vi "CAN.vi"() -> ()   [LabVIEW 2020]
uses:
  Global_Variable/Global.vi
  Global_Variable/A180648.vi
  Libraries/ZLG_CAN/ZLG_CAN.lvlib
panel:
  out "error out":errorcluster caption="错误输出"
  in  "CAN 通道":u32(ring) items=["0", "1"]
  in  "索引":u32(ring) items=["0", "1", "2", "3", "4", "5", "6", "7", "8"]
  in  "设备类型":u32(ring)=27 items=["PCI5121"=1, "PCI9810"=2, "USBCAN1"=3, "USBCAN2"=4, "PCI9820"=5, "PCI5110"=7, "PC104CAN"=11, "CANETUDP"=12, "PCI9840B"=14, "PC104C2"=15, "PCI9820I"=16, "CANETTCP"=17, "PCIE9221"=24, "PCI5010U"=19, "USBCAN_E_U"=20, "USBCAN_2E_U"=21, "PCI5020U"=22, "PCIE9120I"=27, "PCIE9110I"=28, "PCIE9140I"=29]
  in  "Stop":bool
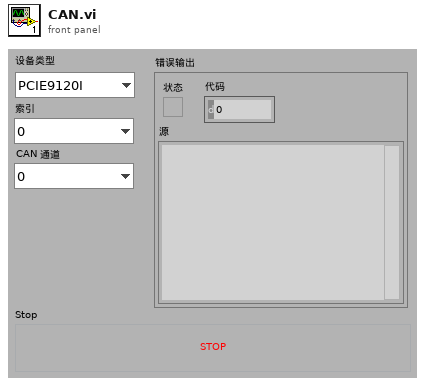
[diagram p1: front panel]
types:
  T1 = cluster{"波特率":u32, "ID":u32, "帧类型":enum8{"标准帧", "扩展帧"}, "帧格式":enum16{"数据帧", "远程帧"}, "周期(ms)":u32}
  T2 = typedef "ZLG_CAN.lvlib/Start_CAN (Reply Payload)--cluster.ctl" = cluster{"Success":bool, "Start_CAN_error":errorcluster}
  T3 = cluster{u8, u8, "y":u8, "y":u8, "y":u8, "y":u8, "y":u8, "y":u8}
  T4 = cluster{"y":u8, "y":u8, "y":u8, u8, u8, "y":u8, "y":u8, "y":u8}
  T5 = cluster{"[0]":u8, "[1]":u8, "[2]":u8, "[3]":u8, "[4]":u8, "[5]":u8, "[6]":u8, "[7]":u8}
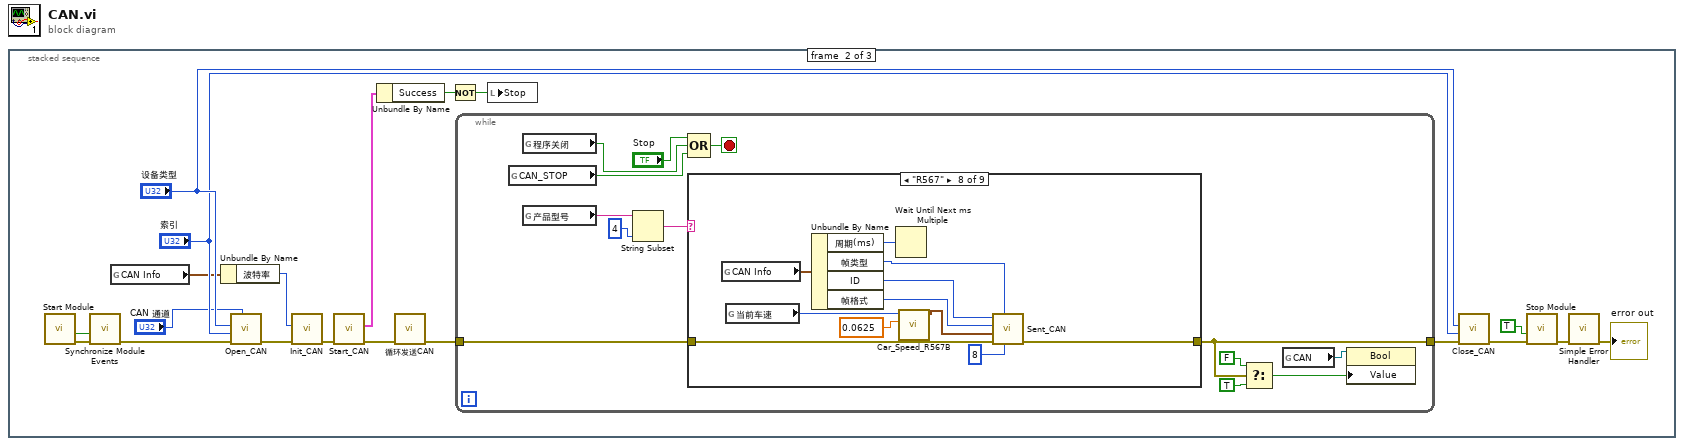
[diagram p0: block diagram]
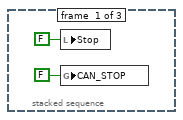
[diagram p2: hidden frame]
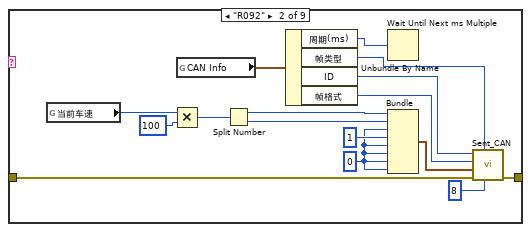
[diagram p4: hidden frame]
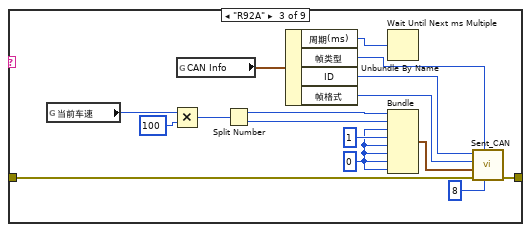
[diagram p5: hidden frame]
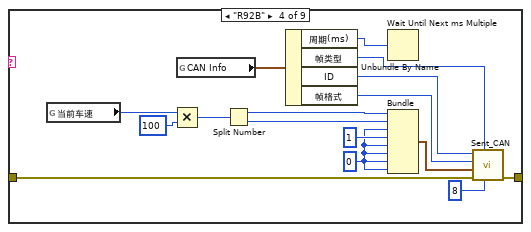
[diagram p6: hidden frame]
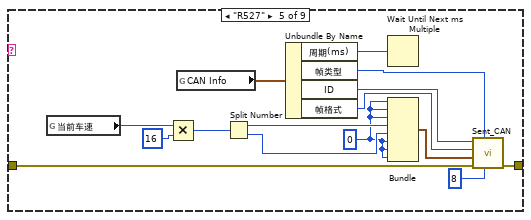
[diagram p7: hidden frame]
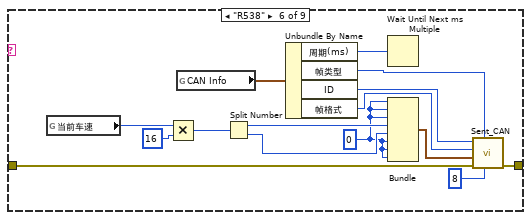
[diagram p8: hidden frame]
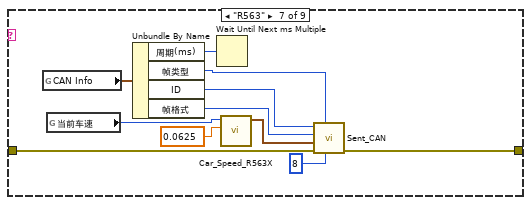
[diagram p9: hidden frame]
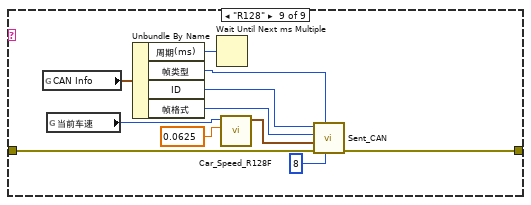
[diagram p10: hidden frame]
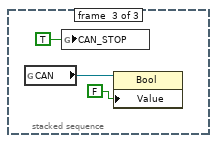
[diagram p11: hidden frame]
diagram:
  n1 = stacked-sequence {
    frame #0 {
      n2 = local write "Stop"(FALSE ("Stop")) -> ()
      n3 = global write "Global.vi" "CAN_STOP"(FALSE ("CAN_STOP")) -> ()
    }
    frame #1 {
      n4 = call "Start Module.vi"() -> ("error out"=w22:errorcluster, "Wait for Event Sync?"=w21:bool)  [unwired: 8 in, 2 out]
      n5 = call "Synchronize Module Events.vi"("error in (no error)"=w22, "Wait for Event Sync?"=w21) -> ("error out"=w20:errorcluster)  [unwired: 9 in]
      n6 = global read "Global.vi" "CAN Info"() -> (w11:T1)
      n7 = Unbundle By Name(w11) -> ("波特率"=w12:u32)
      n8 = call "Open_CAN.vi"("CAN 通道"="CAN 通道", "error in (no error)"=w20, "索引"="索引", "设备类型"="设备类型") -> ("error out"=w17:errorcluster)  [unwired: 7 in]
      n9 = call "Init_CAN.vi"("error in (no error)"=w17, "波特率"=w12) -> ("error out"=w13:errorcluster)  [unwired: 9 in]
      n10 = call "Start_CAN.vi"("error in (no error)"=w13) -> ("error out"=w10:errorcluster, "Reply Payload"=w15:T2)  [unwired: 8 in, 1 out]
      n11 = Unbundle By Name(w15) -> ("Success"=w14:bool)
      n12 = call "循环发送CAN.vi"("错误输入"=w10) -> ("错误输出"=w9:errorcluster)  [unwired: 10 in]
      n13 = Not(x=w14) -> (.not. x?=w8:bool)
      n14 = while {
        tunnel: w9 -> [w27]
        tunnel: [w23] -> w5
        stop <- w34 stop-if-true
        n15 = global read "Global.vi" "CAN_STOP"() -> (w29:bool)
        n16 = global read "Global.vi" "程序关闭"() -> (w33:bool)
        n17 = global read "Global.vi" "产品型号"() -> (w32:string)
        n18 = String Subset(string=w32, length (rest)=4 ("长度（剩余）")) -> (substring=w30:string)  [unwired: 1 in]
        n19 = Compound Arithmetic op=OR ("复合运算")("Stop", w33, w29) -> (w34:bool)
        n20 = case shown="\"R567\"" w30 {
          tunnel: w27 -> [w36 w52 w68 w84 w99 w114 w125 w136 w147]
          tunnel: [w36 w51 w67 w83 w98 w113 w124 w135 w146] -> w23
          frame "假", Default {
          }
          frame "R092" {
            w37 = u8 0 ("y")
            n21 = global read "A180648.vi" "当前车速"() -> (w38:u16)
            n22 = Multiply(x=w38, y=u16 100) -> (x*y=w49:u16)
            n23 = global read "Global.vi" "CAN Info"() -> (w39:T1)
            n24 = Split Number(x=w49) -> (hi(x)=w48:u8, lo(x)=w47:u8)
            n25 = Unbundle By Name(w39) -> ("周期(ms)"=w43:u32, "帧类型"=w41:enum8{"标准帧", "扩展帧"}, "ID"=w40:u32, "帧格式"=w42:enum16{"数据帧", "远程帧"})
            n26 = Wait Until Next ms Multiple(millisecond multiple=w43) -> ()  [unwired: 1 out]
            n27 = Bundle(w48, w47, "y"=w37, "y"=u8 1, "y"=w37, "y"=w37, "y"=w37, "y"=w37) -> (w45:T3)  [unwired: 1 in]
            n28 = call "Sent_CAN.vi"("帧长度"=u8 8, "帧类型"=w41, "error in (no error)"=w52, "帧数据"=w45, "帧格式"=w42, "ID"=w40) -> ("error out"=w51:errorcluster)  [unwired: 5 in]
          }
          frame "R92A" {
            w53 = u8 0 ("y")
            n29 = global read "A180648.vi" "当前车速"() -> (w54:u16)
            n30 = Multiply(x=w54, y=u16 100) -> (x*y=w65:u16)
            n31 = global read "Global.vi" "CAN Info"() -> (w55:T1)
            n32 = Split Number(x=w65) -> (hi(x)=w64:u8, lo(x)=w63:u8)
            n33 = Unbundle By Name(w55) -> ("周期(ms)"=w59:u32, "帧类型"=w57:enum8{"标准帧", "扩展帧"}, "ID"=w56:u32, "帧格式"=w58:enum16{"数据帧", "远程帧"})
            n34 = Wait Until Next ms Multiple(millisecond multiple=w59) -> ()  [unwired: 1 out]
            n35 = Bundle(w64, w63, "y"=w53, "y"=u8 1, "y"=w53, "y"=w53, "y"=w53, "y"=w53) -> (w61:T3)  [unwired: 1 in]
            n36 = call "Sent_CAN.vi"("帧长度"=u8 8, "帧类型"=w57, "error in (no error)"=w68, "帧数据"=w61, "帧格式"=w58, "ID"=w56) -> ("error out"=w67:errorcluster)  [unwired: 5 in]
          }
          frame "R92B" {
            w69 = u8 0 ("y")
            n37 = global read "A180648.vi" "当前车速"() -> (w70:u16)
            n38 = Multiply(x=w70, y=u16 100) -> (x*y=w81:u16)
            n39 = global read "Global.vi" "CAN Info"() -> (w71:T1)
            n40 = Split Number(x=w81) -> (hi(x)=w80:u8, lo(x)=w79:u8)
            n41 = Unbundle By Name(w71) -> ("周期(ms)"=w75:u32, "帧类型"=w73:enum8{"标准帧", "扩展帧"}, "ID"=w72:u32, "帧格式"=w74:enum16{"数据帧", "远程帧"})
            n42 = Wait Until Next ms Multiple(millisecond multiple=w75) -> ()  [unwired: 1 out]
            n43 = Bundle(w80, w79, "y"=w69, "y"=u8 1, "y"=w69, "y"=w69, "y"=w69, "y"=w69) -> (w77:T3)  [unwired: 1 in]
            n44 = call "Sent_CAN.vi"("帧长度"=u8 8, "帧类型"=w73, "error in (no error)"=w84, "帧数据"=w77, "帧格式"=w74, "ID"=w72) -> ("error out"=w83:errorcluster)  [unwired: 5 in]
          }
          frame "R527" {
            w85 = u8 0 ("y")
            n45 = global read "A180648.vi" "当前车速"() -> (w88:u16)
            n46 = Multiply(x=w88, y=u16 16) -> (x*y=w96:u16)
            n47 = global read "Global.vi" "CAN Info"() -> (w89:T1)
            n48 = Split Number(x=w96) -> (hi(x)=w87:u8, lo(x)=w86:u8)
            n49 = Unbundle By Name(w89) -> ("周期(ms)"=w93:u32, "帧类型"=w91:enum8{"标准帧", "扩展帧"}, "ID"=w90:u32, "帧格式"=w92:enum16{"数据帧", "远程帧"})
            n50 = Wait Until Next ms Multiple(millisecond multiple=w93) -> ()  [unwired: 1 out]
            n51 = Bundle("y"=w85, "y"=w85, "y"=w85, w87, w86, "y"=w85, "y"=w85, "y"=w85) -> (w95:T4)  [unwired: 1 in]
            n52 = call "Sent_CAN.vi"("帧长度"=u8 8, "帧类型"=w91, "error in (no error)"=w99, "帧数据"=w95, "帧格式"=w92, "ID"=w90) -> ("error out"=w98:errorcluster)  [unwired: 5 in]
          }
          frame "R538" {
            w100 = u8 0 ("y")
            n53 = global read "A180648.vi" "当前车速"() -> (w103:u16)
            n54 = Multiply(x=w103, y=u16 16) -> (x*y=w111:u16)
            n55 = global read "Global.vi" "CAN Info"() -> (w104:T1)
            n56 = Split Number(x=w111) -> (hi(x)=w102:u8, lo(x)=w101:u8)
            n57 = Unbundle By Name(w104) -> ("周期(ms)"=w108:u32, "帧类型"=w106:enum8{"标准帧", "扩展帧"}, "ID"=w105:u32, "帧格式"=w107:enum16{"数据帧", "远程帧"})
            n58 = Wait Until Next ms Multiple(millisecond multiple=w108) -> ()  [unwired: 1 out]
            n59 = Bundle("y"=w100, "y"=w100, "y"=w100, w102, w101, "y"=w100, "y"=w100, "y"=w100) -> (w110:T4)  [unwired: 1 in]
            n60 = call "Sent_CAN.vi"("帧长度"=u8 8, "帧类型"=w106, "error in (no error)"=w114, "帧数据"=w110, "帧格式"=w107, "ID"=w105) -> ("error out"=w113:errorcluster)  [unwired: 5 in]
          }
          frame "R563" {
            n61 = global read "Global.vi" "CAN Info"() -> (w118:T1)
            n62 = global read "A180648.vi" "当前车速"() -> (w116:u16)
            n63 = Unbundle By Name(w118) -> ("周期(ms)"=w122:u32, "帧类型"=w120:enum8{"标准帧", "扩展帧"}, "ID"=w119:u32, "帧格式"=w121:enum16{"数据帧", "远程帧"})
            n64 = Wait Until Next ms Multiple(millisecond multiple=w122) -> ()  [unwired: 1 out]
            n65 = call "Car_Speed_R563X.vi"("精度"=0.0625, "车速"=w116) -> ("报文"=w115:T5)  [unwired: 9 in]
            n66 = call "Sent_CAN.vi"("帧长度"=u8 8, "帧类型"=w120, "error in (no error)"=w125, "帧数据"=w115, "帧格式"=w121, "ID"=w119) -> ("error out"=w124:errorcluster)  [unwired: 5 in]
          }
          frame "R567" {
            n67 = global read "Global.vi" "CAN Info"() -> (w129:T1)
            n68 = global read "A180648.vi" "当前车速"() -> (w128:u16)
            n69 = Unbundle By Name(w129) -> ("周期(ms)"=w133:u32, "帧类型"=w131:enum8{"标准帧", "扩展帧"}, "ID"=w130:u32, "帧格式"=w132:enum16{"数据帧", "远程帧"})
            n70 = Wait Until Next ms Multiple(millisecond multiple=w133) -> ()  [unwired: 1 out]
            n71 = call "Car_Speed_R567B.vi"("精度"=0.0625, "车速"=w128) -> ("报文"=w126:T5)  [unwired: 9 in]
            n72 = call "Sent_CAN.vi"("帧长度"=u8 8, "帧类型"=w131, "error in (no error)"=w136, "帧数据"=w126, "帧格式"=w132, "ID"=w130) -> ("error out"=w135:errorcluster)  [unwired: 5 in]
          }
          frame "R128" {
            n73 = global read "Global.vi" "CAN Info"() -> (w140:T1)
            n74 = global read "A180648.vi" "当前车速"() -> (w138:u16)
            n75 = Unbundle By Name(w140) -> ("周期(ms)"=w144:u32, "帧类型"=w142:enum8{"标准帧", "扩展帧"}, "ID"=w141:u32, "帧格式"=w143:enum16{"数据帧", "远程帧"})
            n76 = Wait Until Next ms Multiple(millisecond multiple=w144) -> ()  [unwired: 1 out]
            n77 = call "Car_Speed_R128F.vi"("精度"=0.0625, "车速"=w138) -> ("报文"=w139:T5)  [unwired: 9 in]
            n78 = call "Sent_CAN.vi"("帧长度"=u8 8, "帧类型"=w142, "error in (no error)"=w147, "帧数据"=w139, "帧格式"=w143, "ID"=w141) -> ("error out"=w146:errorcluster)  [unwired: 5 in]
          }
        }
        n79 = Select(t=FALSE, s=w23, f=TRUE) -> (s? t:f=w24:bool)
        n80 = global read "Global.vi" "CAN"() -> (w28:refnum<vi>)
        n81 = property class="Bool"(reference=w28, "Value"=w24) -> ()  [unwired: 1 in, 2 out]
      }
      n82 = local write "Stop"(w8) -> ()
      n83 = call "Close_CAN.vi"("error in (no error)"=w5, "索引"="索引", "设备类型"="设备类型") -> ("error out"=w6:errorcluster)  [unwired: 8 in]
      n84 = call "Stop Module.vi"("error in (no error)"=w6, "Wait for Module to Stop? (F)"=TRUE) -> ("error out"=w4:errorcluster)  [unwired: 9 in]
      n85 = call <vilib>:"Simple Error Handler.vi"("error in (no error)"=w4) -> ("error out"=→"error out":errorcluster)  [unwired: 4 in, 4 out]
    }
    frame #2 {
      n86 = global read "Global.vi" "CAN"() -> (w149:refnum<vi>)
      n87 = global write "Global.vi" "CAN_STOP"(TRUE ("CAN_STOP")) -> ()
      n88 = property class="Bool"(reference=w149, "Value"=FALSE) -> ()  [unwired: 1 in, 2 out]
    }
  }
